vi "Load System Properties UI.vi"(8 "error in (no error)":errorcluster, 11 "Editor Handler out":refnum<class "Imager Handler.lvclass">) -> (0 "error out":errorcluster, 3 "VI out":refnum<vi>)   [LabVIEW 2016]
uses:
  Imager Handler.lvclass
  System Properties UI.vi
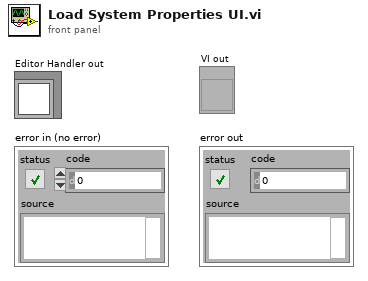
[diagram p1: front panel]
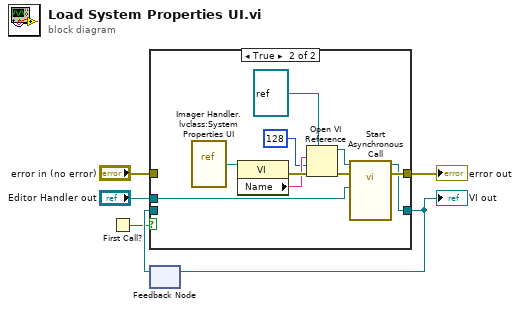
[diagram p0: block diagram]
diagram:
  n1 = First Call?() -> (First Call?: T/F=w2:bool)
  n2 = feedback #1() -> (w3:refnum<vi>)  [unwired: 1 in]
  n3 = case shown="True" w2 {
    tunnel: "error in (no error)" -> [w7 _]
    tunnel: [w7 w10] -> w5
    tunnel: [w8 w9] -> w4
    tunnel: w3 -> [w8 _]
    tunnel: "Editor Handler out" -> [_ w13]
    frame False {
    }
    frame True {
      n4 = vi-ref "Imager Handler.lvclass:System Properties UI.vi"() -> (w16:refnum<vi>)
      n5 = property class="VI"(reference=w16) -> (error out=w18:errorcluster, "Name"=w17:string)  [unwired: 1 in, 1 out]
      n6 = Open VI Reference(type specifier VI Refnum (for type only)=refnum<vi> refnum, vi path=w17, options=128, error in (no error)=w18) -> (vi reference=w15:refnum<vi>, error out=w11:errorcluster)  [unwired: 2 in]
      n7 = call-by-ref "Start Asynchronous Call"(reference=w15, error in=w11, "Editor Handler in"=w13) -> (reference out=w9:refnum<vi>, error out=w10:errorcluster)  [unwired: 9 in, 2 out]
    }
  }
  "error out" <- w5
  "VI out" <- w4
  n8 = feedback-in #1(w4) -> ()
